vi "CRYInsert Socket.vi"(5 "sOption2":string, 6 "Step No.":i32=-1, 7 "sOption1":string, 8 "Waves":T1 {"Y dB ref" format="%.1f"; "Y axis" items=["Log", "Lin"]; "Y data" items=["dB", "Lin"]; "X data" items=["dB", "Lin"]}, 9 "Results":T5 {"Margin" format="%.2f"}, 10 "Values":T3 {"Z data" items=["dB", "Lin"]; "X data" items=["dB", "Lin"]; "Y data" items=["dB", "Lin"]; "Z dB ref" format="%.1f"; "Z axis" items=["Log", "Lin"]; "X dB ref" format="%.1f"; "X axis" items=["Log", "Lin"]; "Y axis" items=["Log", "Lin"]; "Y dB ref" format="%.1f"; "Curve"."z" format="%.2f"; "Curve"."y" format="%.2f"; "Curve"."x" format="%.2f"}, 11 "Curves":T3 {"Z data" items=["dB", "Lin"]; "X data" items=["dB", "Lin"]; "Y data" items=["dB", "Lin"]; "Z dB ref" format="%.1f"; "Z axis" items=["Log", "Lin"]; "X dB ref" format="%.1f"; "X axis" items=["Log", "Lin"]; "Y axis" items=["Log", "Lin"]; "Y dB ref" format="%.1f"; "Curve"."z" format="%.2f"; "Curve"."y" format="%.2f"; "Curve"."x" format="%.2f"}) -> (3 "Inserted Names Out":string[](array[string]))   [LabVIEW 2013]
uses:
  CRYSystem/Typedef Control/CRYData Cluster Array.ctl
  CRYSystem/Typedef Control/CRYData Cluster.ctl
  CRYSystem/Typedef Control/CRYResult Cluster Array.ctl
  CRYSystem/Typedef Control/CRYResult Cluster.ctl
  CRYSystem/Typedef Control/CRYWaveform Cluster Array.ctl
  CRYSystem/Typedef Control/CRYWaveform Cluster.ctl
  Global/CRYCurve Library Global.vi
  Global/CRYCurves Array Global.vi
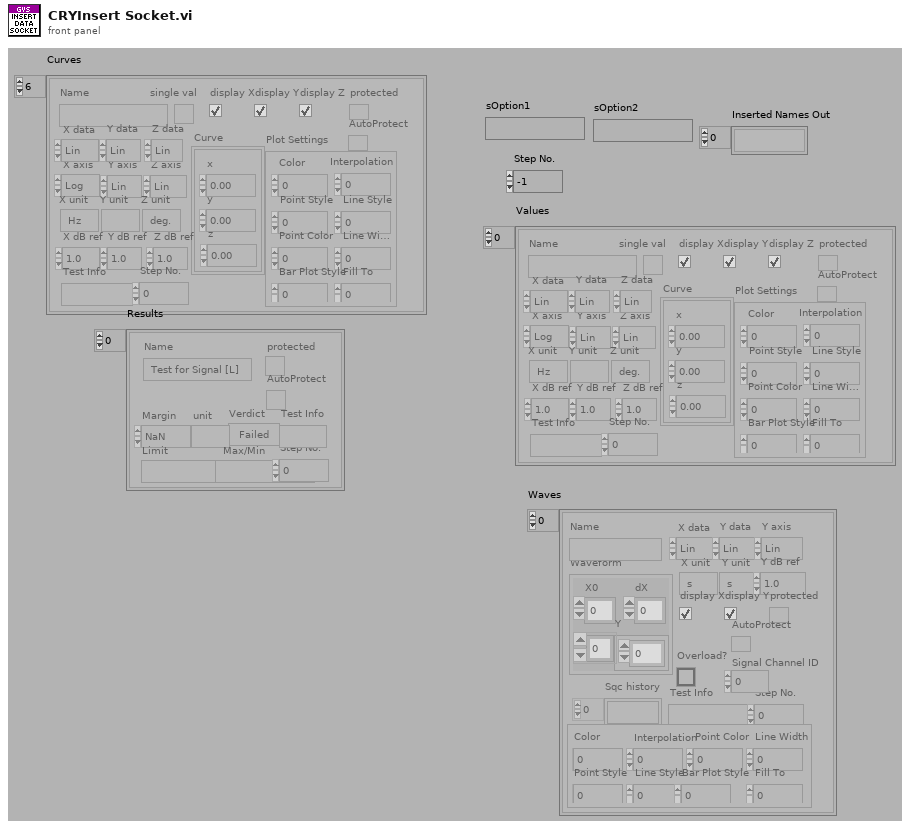
[diagram p1: front panel]
types:
  T1 = typedef "CRYWaveform Cluster Array.ctl" = T2[]
  T2 = typedef "CRYWaveform Cluster.ctl" = cluster{"Waveform":cluster{"X0":dbl, "dX":dbl, "Y":sgl[]}, "X data":u16, "Y data":u16, "Y axis":u16, "X unit":string, "Y unit":string, "Y dB ref":dbl, "display Y":bool, "display X":bool, "Overload?":bool, "Test Info":string, "Step No.":i32, "Name":string, "protected":bool, "Sqc history":string[], "Signal Channel ID":i32, "Plot Settings":cluster{"Color":u32, "Interpolation":u8, "Point Style":u8, "Line Style":u8, "Point Color":u32, "Line Width":u8, "Bar Plot Style":u8, "Fill To":i16}, "AutoProtect":bool}
  T3 = typedef "CRYData Cluster Array.ctl" = T4[]
  T4 = typedef "CRYData Cluster.ctl" = cluster{"Name":string, "Curve":cluster{"x":dbl, "y":dbl, "z":dbl}[], "X data":u16, "Y data":u16, "Z data":u16, "X axis":u16, "Y axis":u16, "Z axis":u16, "X unit":string, "Y unit":string, "Z unit":string, "X dB ref":dbl, "Y dB ref":dbl, "Z dB ref":dbl, "single val":bool, "protected":bool, "display X":bool, "display Y":bool, "display Z":bool, "Test Info":string, "Step No.":i32, "Plot Settings":cluster{"Color":u32, "Interpolation":u8, "Point Style":u8, "Line Style":u8, "Point Color":u32, "Line Width":u8, "Bar Plot Style":u8, "Fill To":i16}, "AutoProtect":bool}
  T5 = typedef "CRYResult Cluster Array.ctl" = T6[]
  T6 = typedef "CRYResult Cluster.ctl" = cluster{"Name":string, "Margin":dbl, "unit":string, "Verdict":bool, "Limit":string, "Max/Min":string, "protected":bool, "Step No.":i32, "Test Info":string, "AutoProtect":bool}
  T7 = cluster{"CurveOld":string[], "ValueOld":string[], "ResultOld":string[], "WFMOld":string[], "CurveNew":string[], "ValueNew":string[], "ResultNew":string[], "WFMNew":string[]}
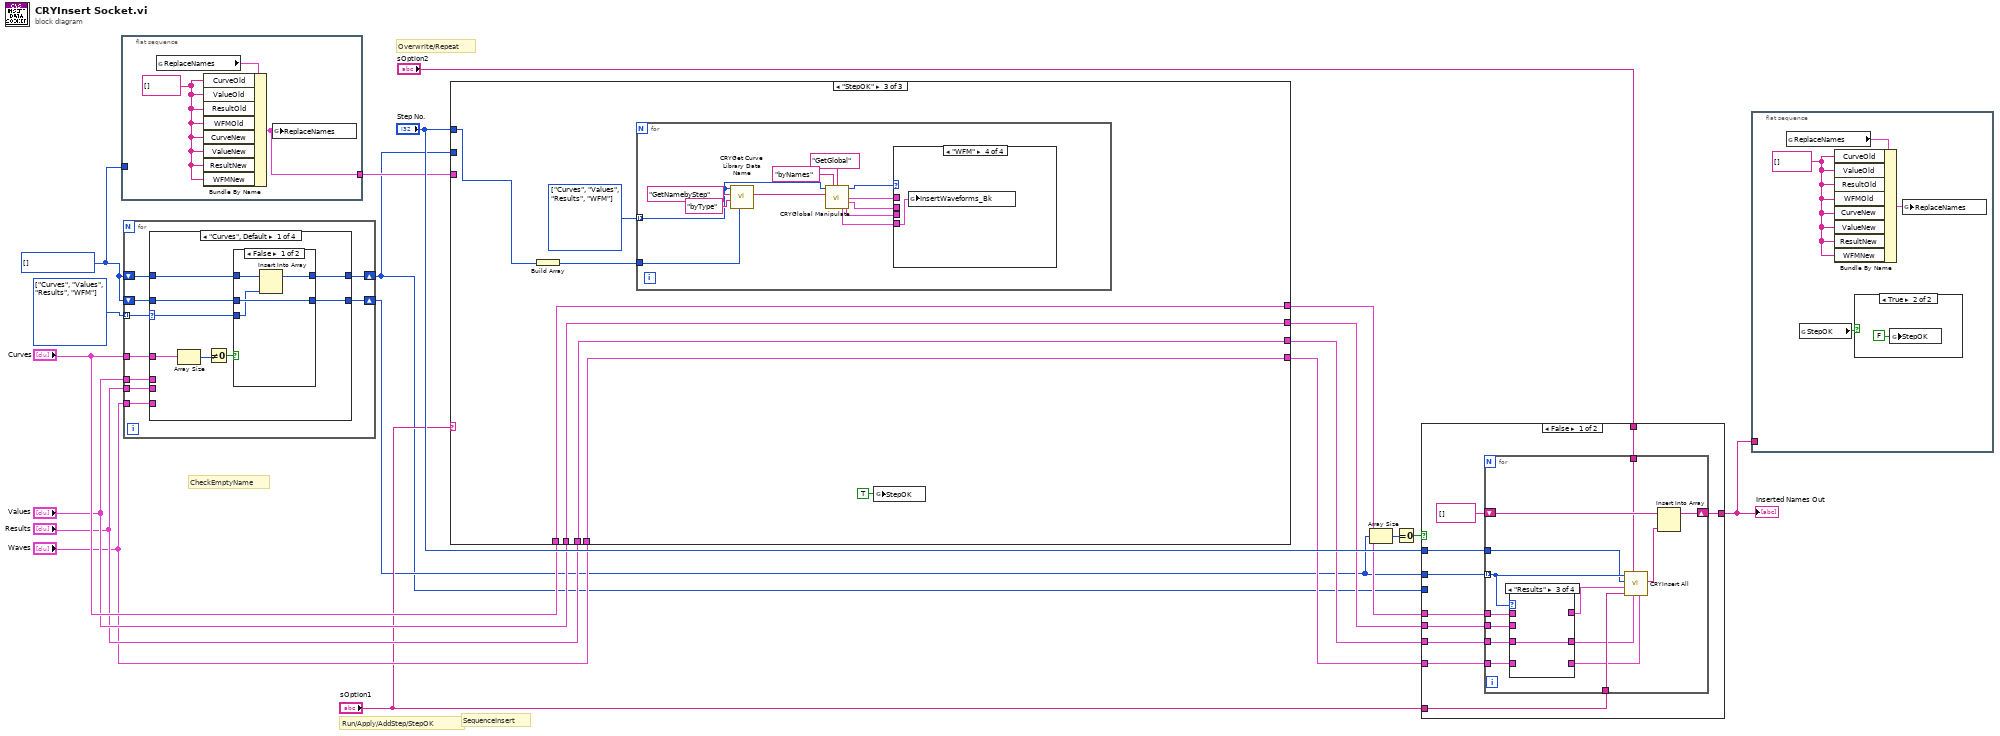
[diagram p0: block diagram]
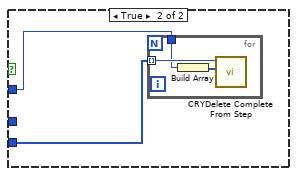
[diagram p5: hidden frame]
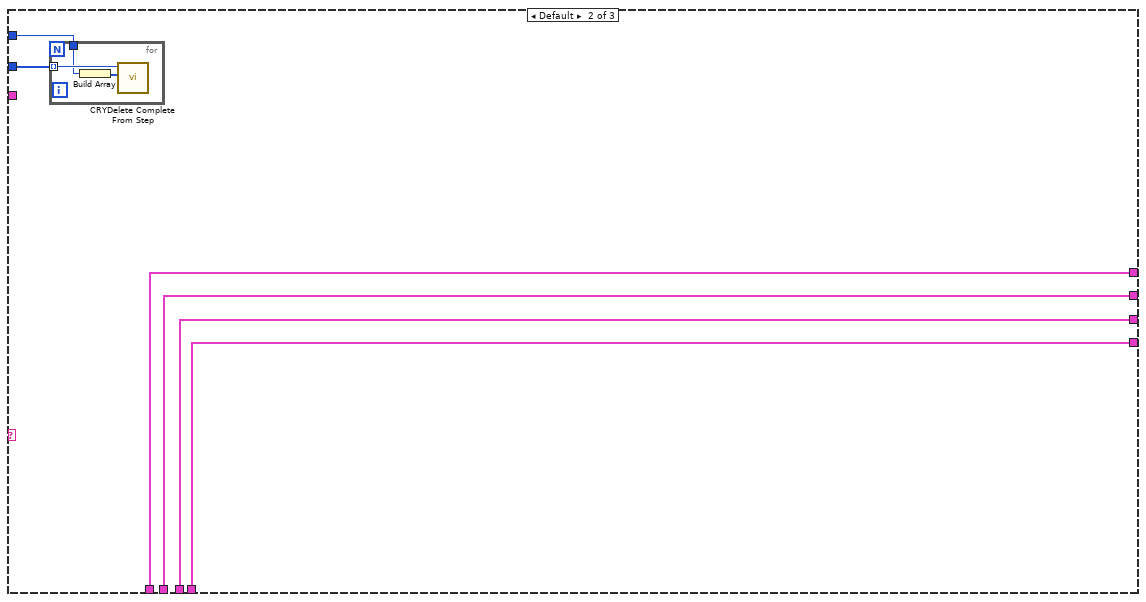
[diagram p8: hidden frame]
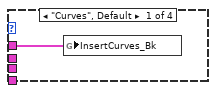
[diagram p9: hidden frame]
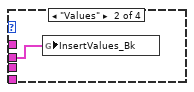
[diagram p10: hidden frame]
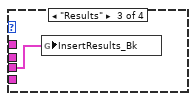
[diagram p11: hidden frame]
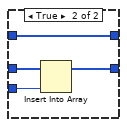
[diagram p12: hidden frame]
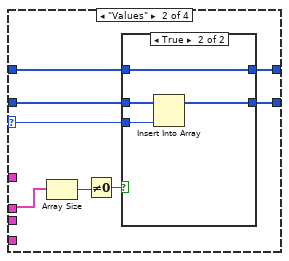
[diagram p13: hidden frame]
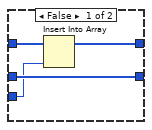
[diagram p14: hidden frame]
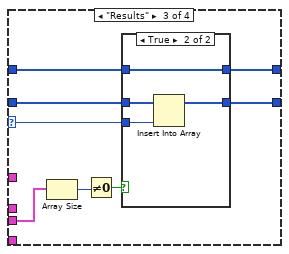
[diagram p15: hidden frame]
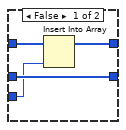
[diagram p16: hidden frame]
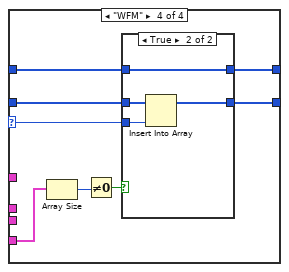
[diagram p17: hidden frame]
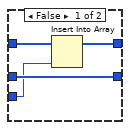
[diagram p18: hidden frame]
diagram:
  w7 = enum16{"Curves", "Values", "Results", "WFM"}[] [] items=["Curves", "Values", "Results", "WFM"]
  w17 = enum16{"Curves", "Values", "Results", "WFM"}[] [enum."Curves", enum."Values", enum."Results", enum."WFM"] items=["Curves", "Values", "Results", "WFM"]
  # "CheckEmptyName"
  # "SequenceInsert"
  # "Run/Apply/AddStep/StepOK"
  # "Overwrite/Repeat"
  n1 = flat-sequence {
    tunnel: w7 -> [_]
    tunnel: [w20] -> w6
    frame #0 {
      w21 = string[] [] ("CurveOld")
      n2 = global read "CRYCurve Library Global.vi" "ReplaceNames"() -> (w22:T7)
      n3 = Bundle By Name(cluster=w22, "CurveOld"=w21, "ValueOld"=w21, "ResultOld"=w21, "WFMOld"=w21, "CurveNew"=w21, "ValueNew"=w21, "ResultNew"=w21, "WFMNew"=w21) -> (w20:T7)
      n4 = global write "CRYCurve Library Global.vi" "ReplaceNames"(w20) -> ()
    }
  }
  n5 = for {
    tunnel: w17 -> [w31] mode=indexing
    tunnel: "Curves" -> [w30]
    shift-right: [w29] -> w4
    shift-left: w7 -> [w28]
    shift-right: [w27] -> w1
    shift-left: w7 -> [w26]
    tunnel: "Values" -> [w25]
    tunnel: "Results" -> [w24]
    tunnel: "Waves" -> [w23]
    n6 = case shown="\"Curves\", Default" w31 {
      selector: w31 -> [w36 w53 w69 w85]
      tunnel: w30 -> [w37 _ _ _]
      tunnel: [w35 w52 w68 w84] -> w29
      tunnel: w28 -> [w34 w51 w67 w83]
      tunnel: [w33 w50 w66 w82] -> w27
      tunnel: w26 -> [w32 w49 w65 w81]
      tunnel: w25 -> [_ w48 _ _]
      tunnel: w24 -> [_ _ w64 _]
      tunnel: w23 -> [_ _ _ w80]
      frame "Curves", Default {
        n7 = Array Size(array=w37) -> (size(s)=w39:i32)
        n8 = Not Equal To 0?(x=w39) -> (x != 0?=w38:bool)
        n9 = case shown="False" w38 {
          tunnel: w36 -> [w42 w47]
          tunnel: [w43 w46] -> w35
          tunnel: w34 -> [w43 w45]
          tunnel: [w41 w44] -> w33
          tunnel: w32 -> [w40 w44]
          frame False {
            n10 = Insert Into Array(array=w40, new element=w42) -> (w41:enum16{"Curves", "Values", "Results", "WFM"}[])  [unwired: 1 in]
          }
          frame True {
            n11 = Insert Into Array(array=w45, new element=w47) -> (w46:enum16{"Curves", "Values", "Results", "WFM"}[])  [unwired: 1 in]
          }
        }
      }
      frame "Values" {
        n12 = Array Size(array=w48) -> (size(s)=w55:i32)
        n13 = Not Equal To 0?(x=w55) -> (x != 0?=w54:bool)
        n14 = case shown="True" w54 {
          tunnel: w53 -> [w58 w63]
          tunnel: [w59 w62] -> w52
          tunnel: w51 -> [w59 w61]
          tunnel: [w57 w60] -> w50
          tunnel: w49 -> [w56 w60]
          frame False {
            n15 = Insert Into Array(array=w56, new element=w58) -> (w57:enum16{"Curves", "Values", "Results", "WFM"}[])  [unwired: 1 in]
          }
          frame True {
            n16 = Insert Into Array(array=w61, new element=w63) -> (w62:enum16{"Curves", "Values", "Results", "WFM"}[])  [unwired: 1 in]
          }
        }
      }
      frame "Results" {
        n17 = Array Size(array=w64) -> (size(s)=w71:i32)
        n18 = Not Equal To 0?(x=w71) -> (x != 0?=w70:bool)
        n19 = case shown="True" w70 {
          tunnel: w69 -> [w74 w79]
          tunnel: [w75 w78] -> w68
          tunnel: w67 -> [w75 w77]
          tunnel: [w73 w76] -> w66
          tunnel: w65 -> [w72 w76]
          frame False {
            n20 = Insert Into Array(array=w72, new element=w74) -> (w73:enum16{"Curves", "Values", "Results", "WFM"}[])  [unwired: 1 in]
          }
          frame True {
            n21 = Insert Into Array(array=w77, new element=w79) -> (w78:enum16{"Curves", "Values", "Results", "WFM"}[])  [unwired: 1 in]
          }
        }
      }
      frame "WFM" {
        n22 = Array Size(array=w80) -> (size(s)=w87:i32)
        n23 = Not Equal To 0?(x=w87) -> (x != 0?=w86:bool)
        n24 = case shown="True" w86 {
          tunnel: w85 -> [w90 w95]
          tunnel: [w91 w94] -> w84
          tunnel: w83 -> [w91 w93]
          tunnel: [w89 w92] -> w82
          tunnel: w81 -> [w88 w92]
          frame False {
            n25 = Insert Into Array(array=w88, new element=w90) -> (w89:enum16{"Curves", "Values", "Results", "WFM"}[])  [unwired: 1 in]
          }
          frame True {
            n26 = Insert Into Array(array=w93, new element=w95) -> (w94:enum16{"Curves", "Values", "Results", "WFM"}[])  [unwired: 1 in]
          }
        }
      }
    }
  }
  n27 = case shown="\"StepOK\"" "sOption1" {
    tunnel: w1 -> [_ w105 _]
    tunnel: "Step No." -> [_ w104 w116]
    tunnel: "Curves" -> [w99 w103 w115]
    tunnel: "Values" -> [w98 w102 w114]
    tunnel: "Results" -> [w97 w101 w113]
    tunnel: "Waves" -> [w96 w100 w112]
    tunnel: [w99 w103 w115] -> w12
    tunnel: [w98 w102 w114] -> w11
    tunnel: [w97 w101 w113] -> w10
    tunnel: [w96 w100 w112] -> w9
    tunnel: w6 -> [_ _ _]
    frame "Run", "SequenceInsert" {
    }
    frame Default {
      n28 = for {
        tunnel: w105 -> [w108] mode=indexing
        tunnel: w104 -> [w107]
        n29 = Build Array(w107) -> (w106:i32[])
        n30 = call "CRYDelete Complete From Step.vi"("Step No."=w106, "Type In"=w108) -> ()  [unwired: 9 in, 1 out]
      }
    }
    frame "StepOK" {
      w110 = enum16{"Curves", "Values", "Results", "WFM"}[] [enum."Curves", enum."Values", enum."Results", enum."WFM"] items=["Curves", "Values", "Results", "WFM"]
      n31 = Build Array(w116) -> (w109:i32[])
      n32 = for {
        tunnel: w110 -> [w125] mode=indexing
        tunnel: w109 -> [w126]
        n33 = call "CRYGet Curve Library Data Name.vi"("nData"=w126, "sOption"="byType", "sAction"="GetNamebyStep", "Type"=w125) -> ("sNames"=w124:string[])  [unwired: 4 in, 3 out]
        n34 = call "CRYGlobal Manipulate.vi"("Type"=w125, "sOption"="byNames", "sAction"="GetGlobal", "sData"=w124) -> ("Type out"=w121:enum16{"Curves", "Values", "Results", "WFM"}, "Curves Out"=w120:T4[], "Values Out"=w119:T4[], "WFM Out"=w117:T2[], "Results Out"=w118:T6[])  [unwired: 5 in, 2 out]
        n35 = case shown="\"WFM\"" w121 {
          tunnel: w120 -> [w129 _ _ _]
          tunnel: w119 -> [_ w130 _ _]
          tunnel: w118 -> [_ _ w131 _]
          tunnel: w117 -> [_ _ _ w132]
          frame "Curves", Default {
            n36 = global write "CRYCurves Array Global.vi" "InsertCurves_Bk"(w129) -> ()
          }
          frame "Values" {
            n37 = global write "CRYCurves Array Global.vi" "InsertValues_Bk"(w130) -> ()
          }
          frame "Results" {
            n38 = global write "CRYCurves Array Global.vi" "InsertResults_Bk"(w131) -> ()
          }
          frame "WFM" {
            n39 = global write "CRYCurves Array Global.vi" "InsertWaveforms_Bk"(w132) -> ()
          }
        }
      }
      n40 = global write "CRYCurve Library Global.vi" "StepOK"(TRUE ("StepOK")) -> ()
    }
  }
  n41 = Array Size(array=w4) -> (size(s)=w5:i32)
  n42 = Equal To 0?(x=w5) -> (x = 0?=w2:bool)
  n43 = case shown="False" w2 {
    tunnel: "sOption2" -> [w142 _]
    tunnel: "Step No." -> [w141 w161]
    tunnel: w12 -> [w139 _]
    tunnel: w11 -> [w138 _]
    tunnel: w10 -> [w137 _]
    tunnel: w9 -> [w136 _]
    tunnel: "sOption1" -> [w135 _]
    tunnel: w4 -> [w134 _]
    tunnel: [w133 _] -> w3
    tunnel: w1 -> [_ w162]
    frame False {
      n44 = for {
        tunnel: w134 -> [w148] mode=indexing
        tunnel: w139 -> [w156]
        tunnel: w136 -> [w153]
        tunnel: w138 -> [w155]
        tunnel: w137 -> [w154]
        shift-right: [w152] -> w133
        shift-left: string[] [] -> [w151]
        tunnel: w135 -> [w150]
        tunnel: w142 -> [w144]
        tunnel: w141 -> [w143]
        n45 = case shown="\"Results\"" w148 {
          tunnel: [w157 w158 _ _] -> w149
          tunnel: w156 -> [w157 _ _ _]
          tunnel: w155 -> [_ w158 _ _]
          tunnel: w154 -> [_ _ w159 _]
          tunnel: w153 -> [_ _ _ w160]
          tunnel: [_ _ w159 _] -> w146
          tunnel: [_ _ _ w160] -> w145
          frame "Curves", Default {
          }
          frame "Values" {
          }
          frame "Results" {
          }
          frame "WFM" {
          }
        }
        n46 = call "CRYInsert All.vi"("Waves"=w145, "Results"=w146, "sOption2"=w144, "sOption1"=w150, "Curves"=w149, "Step No."=w143, "Type In"=w148) -> ("Inserted Names Out"=w147:string[])  [unwired: 3 in, 1 out]
        n47 = Insert Into Array(array=w151, new element=w147) -> (w152:string[])  [unwired: 1 in]
      }
    }
    frame True {
      n48 = for {
        tunnel: w162 -> [w165] mode=indexing
        tunnel: w161 -> [w164]
        n49 = Build Array(w164) -> (w163:i32[])
        n50 = call "CRYDelete Complete From Step.vi"("Step No."=w163, "Type In"=w165) -> ()  [unwired: 9 in, 1 out]
      }
    }
  }
  "Inserted Names Out" <- w3
  n51 = flat-sequence {
    tunnel: w3 -> [_]
    frame #0 {
      w167 = string[] [] ("CurveOld")
      n52 = global read "CRYCurve Library Global.vi" "ReplaceNames"() -> (w169:T7)
      n53 = global read "CRYCurve Library Global.vi" "StepOK"() -> (w166:bool)
      n54 = Bundle By Name(cluster=w169, "CurveOld"=w167, "ValueOld"=w167, "ResultOld"=w167, "WFMOld"=w167, "CurveNew"=w167, "ValueNew"=w167, "ResultNew"=w167, "WFMNew"=w167) -> (w168:T7)
      n55 = case shown="True" w166 {
        frame False {
        }
        frame True {
          n56 = global write "CRYCurve Library Global.vi" "StepOK"(FALSE ("StepOK")) -> ()
        }
      }
      n57 = global write "CRYCurve Library Global.vi" "ReplaceNames"(w168) -> ()
    }
  }
